vi "DisplayResult.vi"(8 "error in (no error)":errorcluster, 10 "Packet Info":T1={"Packet Signature"="", "Sequence Number"=0, "Command"=enum."xml Set LC Input Logic", "Data Message Size"=0, "Data Message Size"="", "Data Message"="", "Error Message Size"=0, "Error Message Size"="", "Error Message"="", "Checksum"=0, "Error Message"={"status"=FALSE, "code"=0, "source"=""}, "Command ID"=""}, 11 "Cluster":T10 {"Parameter"."Expt"."Mass Range"."Resolution Type" items=["High/High", "Medium/Medium", "Low/Low", "High/Medium", "High/Low", "Medium/High", "Medium/Low", "Low/High", "Low/Medium"]}) -> (0 "error in":errorcluster, 3 "Cluster out":T10 {"Parameter"."Expt"."Mass Range"."Resolution Type" items=["High/High", "Medium/Medium", "Low/Low", "High/Medium", "High/Low", "Medium/High", "Medium/Low", "Low/High", "Low/Medium"]})   [LabVIEW 2015]
uses:
  Type/RT Loop Events.ctl
  Type/_RT Parameter.ctl
  Type/_RT Active Ch.ctl
  Type/_RT Expt.ctl
  Type/_Run Mode.ctl
  Type/_RT Mass Range.ctl
  Type/_RT Res Type.ctl
  Type/_RT Command.ctl
  Type/TCP Packet Info.ctl
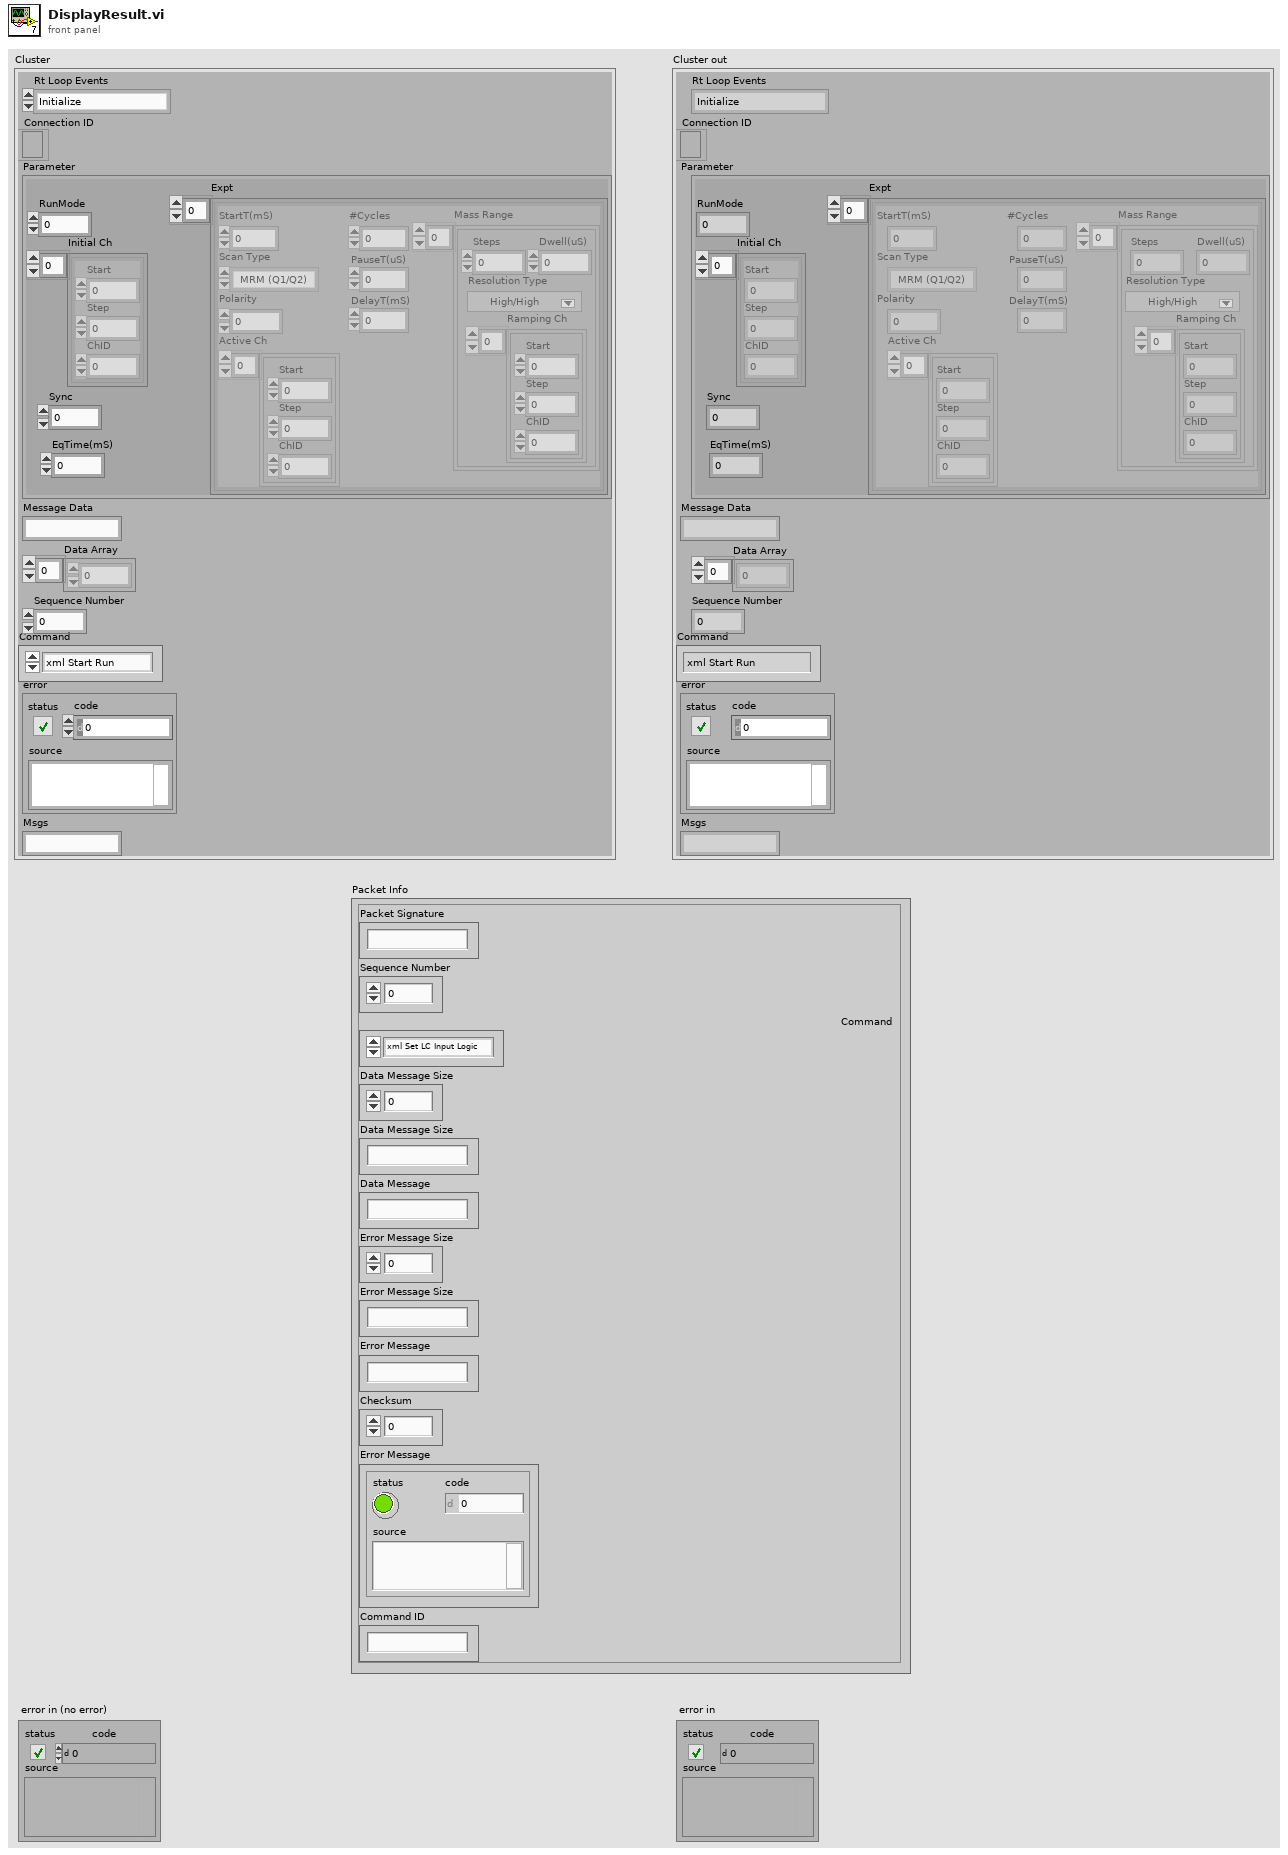
[diagram p1: front panel]
types:
  T1 = typedef "TCP Packet Info.ctl" = cluster{"Packet Signature":string, "Sequence Number":i32, "Command":T2, "Data Message Size":u32, "Data Message Size":string, "Data Message":string, "Error Message Size":u32, "Error Message Size":string, "Error Message":string, "Checksum":u32, "Error Message":errorcluster, "Command ID":string}
  T2 = typedef "_RT Command.ctl" = enum16{"xml Start Run", "xml Start Actual Run", "xml Stop Run", "xml Runtime Update", "xml Get Status", "xml Get Table", "xml Set Table", "xml Get Configuration", "xml System Status", "xml Set LC Input Logic", "xml Get Data", "xml Get Info", "Start", "StartActualRun", "Stop", "Runtime Update", "Get Data", "Get Info", "Get Status", "Get Param", "Get Config", "Get Table", "Read ADC", "Set Oscillator", "Update Config", "Update Table", "Set All Pol", "Set Pol and DC", "Set Max Mass", "Toggle RP", "Toggle EL", "Set PIC", "Initialize Turbo", "Send Turbo Comm", "Close Turbo", "P1", "P2", "P3", "Send Serial", "Set LC Out", "Get LC In", "Read VAC", "Test Table", "Toggle Power", "Get Startup", "Set Startup", "Get ADC Table", "Set ADC Table", "Get Brief Status", "Get Detail Status", "Auxiliary Update", "Set CC Logics", "Set CC Input Logics", "Ignore Error", "invalid"}
  T3 = typedef "RT Loop Events.ctl" = enum16{"Initialize", "Wait for Connection", "Wait for Command", "Send Reply"}
  T4 = typedef "_RT Parameter.ctl" = cluster{"RunMode":i32, "Initial Ch":T5[], "Sync":u8, "Expt":T6[], "EqTime(mS)":i32}
  T5 = typedef "_RT Active Ch.ctl" = cluster{"Start":i32, "Step":i32, "ChID":i32}
  T6 = typedef "_RT Expt.ctl" = cluster{"StartT(mS)":i32, "#Cycles":i32, "Scan Type":T7, "PauseT(uS)":i32, "Polarity":u8, "DelayT(mS)":i32, "Active Ch":T5[], "Mass Range":T8[]}
  T7 = typedef "_Run Mode.ctl" = enum16{"MRM (Q1/Q2)", "Q1 Scan", "Q1 SRM", "Q2 Scan", "Q2 SRM", "Product Scan", "Precursor Scan", "Neutral Loss", "Neutral Gain"}
  T8 = typedef "_RT Mass Range.ctl" = cluster{"Steps":i32, "Dwell(uS)":i32, "Resolution Type":T9, "Ramping Ch":T5[]}
  T9 = typedef "_RT Res Type.ctl" = u16
  T10 = cluster{"Rt Loop Events":T3, "Connection ID":refnum<k5>, "Parameter":T4, "Message Data":string, "Data Array":i32[], "Sequence Number":i32, "Command":T2, "error":errorcluster, "Msgs":string}
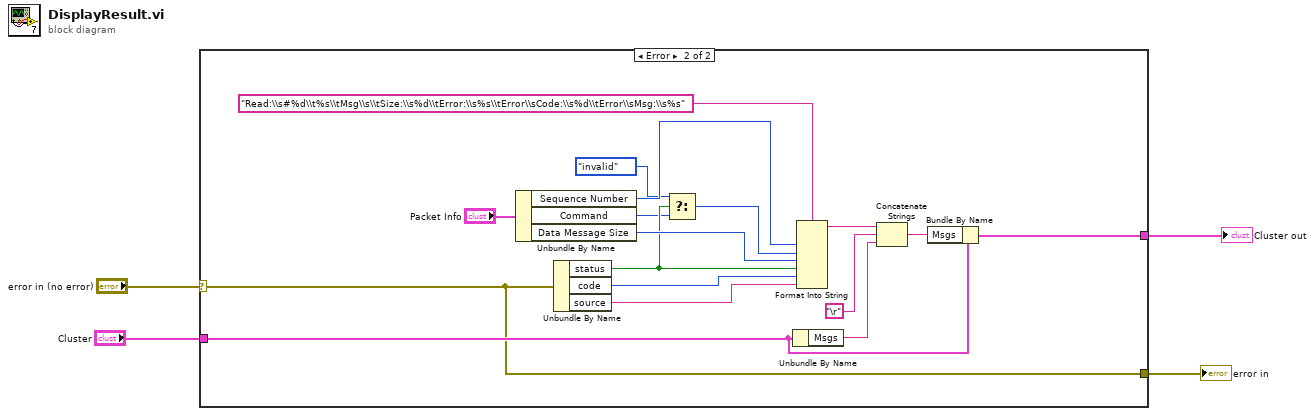
[diagram p0: block diagram]
diagram:
  n1 = case shown="Error" "error in (no error)" {
    selector: "error in (no error)" -> [w6 w7]
    tunnel: "Cluster" -> [w5 w23]
    tunnel: [w5 w22] -> w3
    tunnel: [w6 w7] -> w1
    frame No Error {
    }
    frame Error {
      n2 = Unbundle By Name("Packet Info") -> ("Sequence Number"=w15:i32, "Command"=w9:T2, "Data Message Size"=w14:u32)
      n3 = Unbundle By Name(w7) -> ("status"=w11:bool, "code"=w13:i32, "source"=w12:string)
      n4 = Select(t=_RT_Command."invalid" ("Command"), s=w11, f=w9) -> (s? t:f=w8:T2)
      n5 = Unbundle By Name(w23) -> ("Msgs"=w20:string)
      n6 = Format Into String(format string="Read:\\s#%d\\t%s\\tMsg\\s\\tSize:\\s%d\\tError:\\s%s\\tError\\sCode:\\s%d\\tError\\sMsg:\\s%s", w15, w8, w14, w11, w13, w12) -> (resulting string=w16:string)  [unwired: 2 in, 1 out]
      n7 = Concatenate Strings(w16, "\r", w20) -> (w19:string)
      n8 = Bundle By Name(cluster=w23, "Msgs"=w19) -> (w22:T10)
    }
  }
  "Cluster out" <- w3
  "error in" <- w1
